vi "test_response string.vi"(8 "error in (no error)":errorcluster, 11 "TestCase in":refnum<class "Return Response Triggers.lvclass">) -> (0 "error out":errorcluster, 3 "TestCase out":refnum<class "Return Response Triggers.lvclass">)   [LabVIEW 2017, in "Return Response Triggers.lvclass"]
uses:
  Return Response Triggers.lvclass
  Libraries/SSH/Return Request Configuration.ctl
  Libraries/SSH/Response Configuration.ctl
  Libraries/SSH/Expected Response String Config.ctl
  <vilib>/addons/_JKI Toolkits/VI Tester/TestCase.llb/TestCase.lvclass
  Libraries/SSH/SSH.lvlib
  C:/Program Files (x86)/National Instruments/LabVIEW 2017/vi.lib/addons/_JKI Toolkits/VI Tester/TestCase.llb/TestCase.lvclass
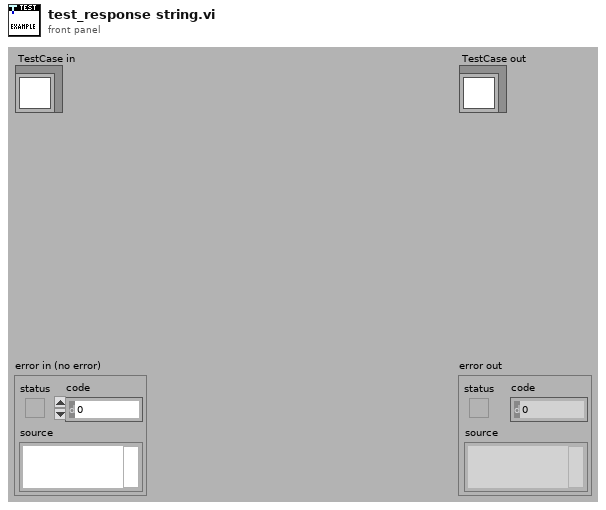
[diagram p1: front panel]
types:
  T1 = typedef "SSH.lvlib/Return Request Configuration.ctl" = cluster{"Response Configuration":T2, "Return Notifier":refnum<notifier>, "Response Requested":bool, "Command":string, "Initial Timer Value":u32}
  T2 = typedef "SSH.lvlib/Response Configuration.ctl" = cluster{"Expected Response String":T3, "Character Count Limit":i32, "Timeout (ms)":i32}
  T3 = typedef "SSH.lvlib/Expected Response String Config.ctl" = cluster{"Expected Response":string, "Search Start Point":enum16{"From Start", "From End"}, "Instance Count":i32}
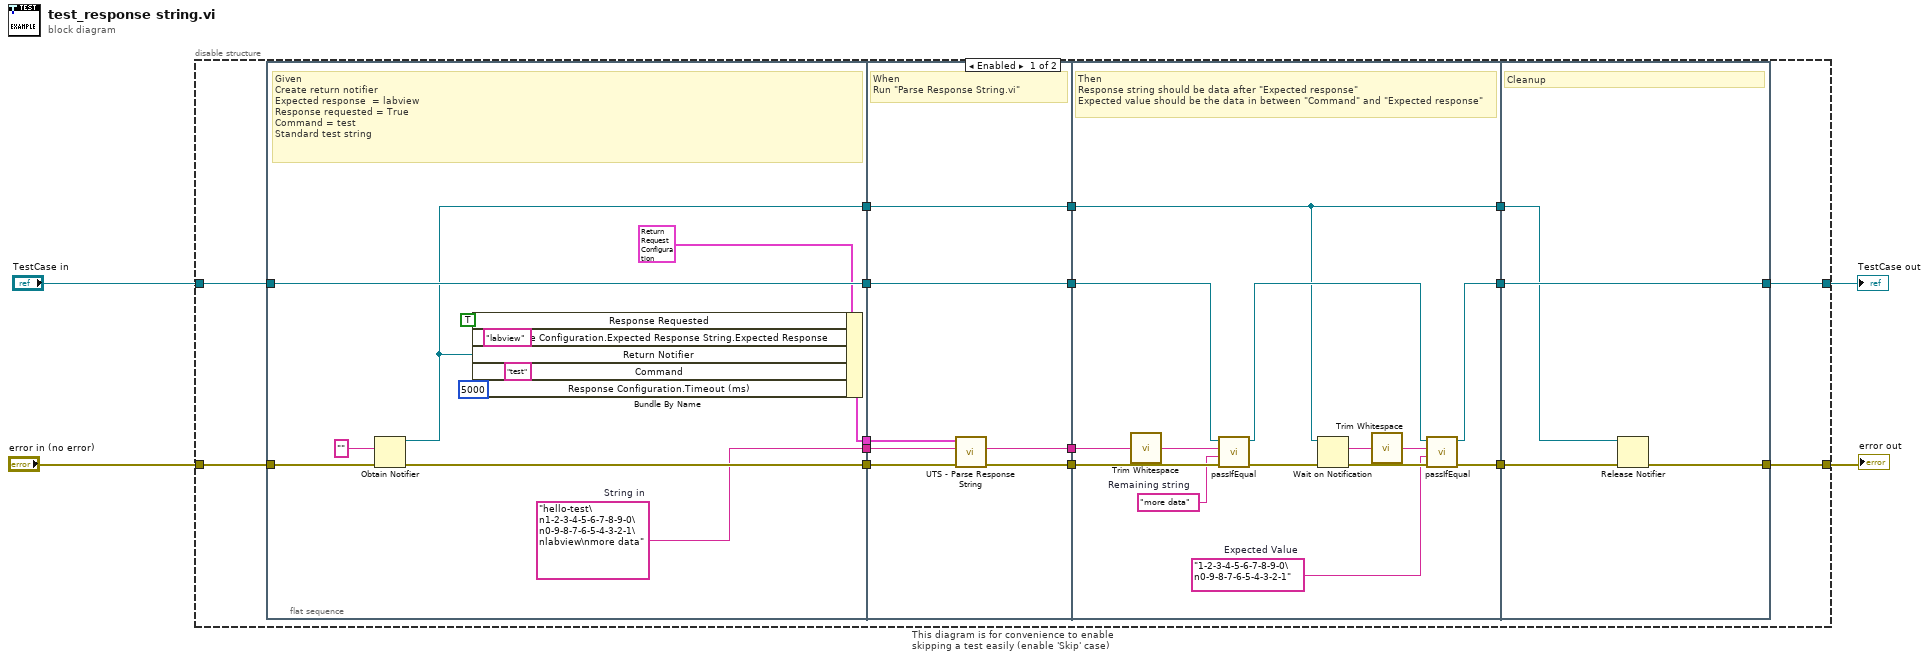
[diagram p0: block diagram]
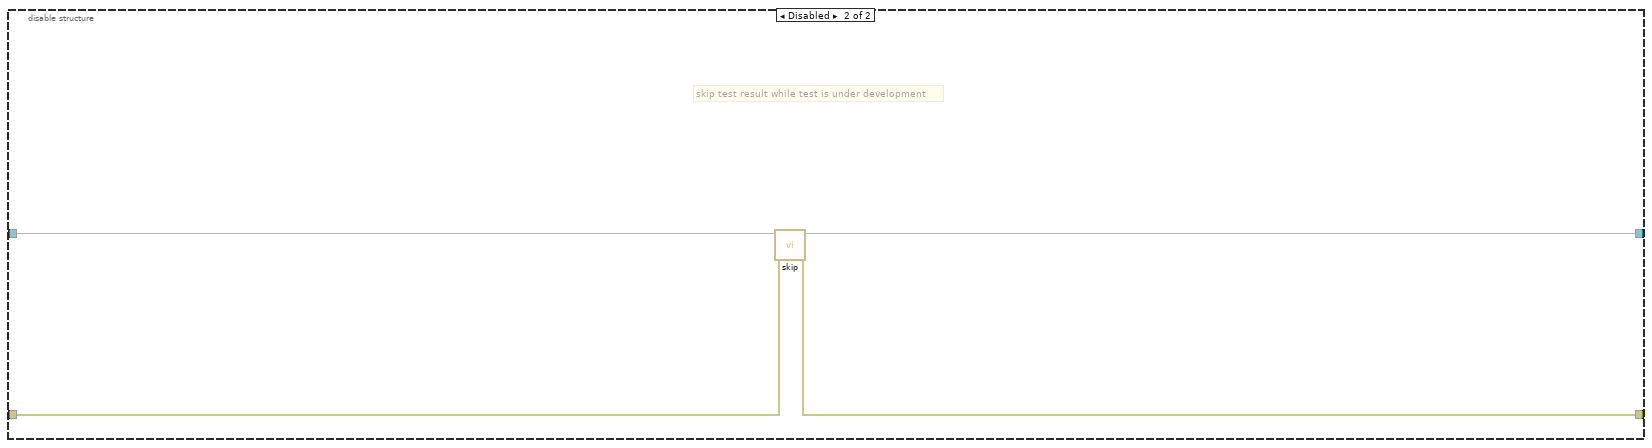
[diagram p2: hidden frame]
diagram:
  n1 = disable-structure "This diagram is for convenience to enable skipping a test easily (enable 'Skip' case)" shown="Enabled" {
    disable-tunnel: "TestCase in" -> [w13 w61]
    disable-tunnel: [w12 w59] -> w1
    disable-tunnel: [w11 w60] -> w3
    disable-tunnel: "error in (no error)" -> [w14 w58]
    frame Enabled {
      n2 = flat-sequence {
        tunnel: w14 -> [w29]
        tunnel: w13 -> [w32]
        tunnel: [w32] -> w20
        tunnel: [w28] -> w19
        tunnel: [w27] -> w10
        tunnel: [w23] -> w9
        tunnel: [w22] -> w8
        tunnel: [w39] -> w18
        tunnel: [w37] -> w17
        tunnel: w20 -> [w39]
        tunnel: w19 -> [w38]
        tunnel: w10 -> [w36]
        tunnel: w9 -> [w33]
        tunnel: w8 -> [w35]
        tunnel: [w34] -> w7
        tunnel: [w33] -> w6
        tunnel: [w46] -> w16
        tunnel: [w48] -> w15
        tunnel: w18 -> [w53]
        tunnel: w17 -> [w52]
        tunnel: w7 -> [w50]
        tunnel: w6 -> [w43]
        tunnel: [w43] -> w5
        tunnel: [w55] -> w11
        tunnel: [w57] -> w12
        tunnel: w16 -> [w57]
        tunnel: w15 -> [w56]
        tunnel: w5 -> [w54]
        frame #0 {
          w22 = "hello-test\n1-2-3-4-5-6-7-8-9-0\n0-9-8-7-6-5-4-3-2-1\nlabview\nmore data"  # String in
          # "Given\nCreate return notifier\nExpected response  = labview\nResponse requested = True\nCommand = test\nStandard test string"
          n3 = Obtain Notifier(notification data type="", error in (no error)=w29) -> (notifier out=w23:refnum<notifier>, error out=w28:errorcluster)  [unwired: 2 in, 1 out]
          n4 = Bundle By Name(cluster=T1 {"Response Configuration"={"Expected Response String"={"Expected Response"="", "Search Start Point"=enum."From Start", "Instance Count"=0}, "Character Count Limit"=0, "Timeout (ms)"=0}, "Return Notifier"=refnum, "Response Requested"=FALSE, "Command"="", "Initial Timer Value"=0} ("Return Request in"), "Response Requested"=TRUE, "Response Configuration.Expected Response String.Expected Response"="labview" ("Response Configuration.Expected Response"), "Return Notifier"=w23, "Command"="test", "Response Configuration.Timeout (ms)"=u32 5000) -> (w27:T1)
        }
        frame #1 {
          # "When\nRun \"Parse Response String.vi\""
          n5 = call "UTS - Parse Response String.vi"("error in (no error)"=w38, "Response String in"=w35, "Return Request in"=w36) -> ("error out"=w37:errorcluster, "Response String out"=w34:string)  [unwired: 6 in, 1 out]
        }
        frame #2 {
          w42 = "more data"  # Remaining string
          w45 = "1-2-3-4-5-6-7-8-9-0\n0-9-8-7-6-5-4-3-2-1"  # Expected Value
          # "Then\nResponse string should be data after \"Expected response\"\nExpected value should be the data in between \"Command\" and \"Expected response\""
          n6 = call <vilib>:"Trim Whitespace.vi"("string"=w50) -> ("trimmed string"=w41:string)  [unwired: 1 in]
          n7 = call-dynamic "passIfEqual.vi"("error in (no error)"=w52, "y"=w42, "x"=w41, "TestCase in"=w53) -> ("error out"=w51:errorcluster, "TestCase out"=w47:refnum<class "Return Response Triggers.lvclass">)  [unwired: 6 in]
          n8 = Wait on Notification(notifier=w43, error in (no error)=w51) -> (notification=w44:string, error out=w49:errorcluster)  [unwired: 2 in, 2 out]
          n9 = call <vilib>:"Trim Whitespace.vi"("string"=w44) -> ("trimmed string"=w40:string)  [unwired: 1 in]
          n10 = call-dynamic "passIfEqual.vi"("error in (no error)"=w49, "y"=w45, "x"=w40, "TestCase in"=w47) -> ("error out"=w48:errorcluster, "TestCase out"=w46:refnum<class "Return Response Triggers.lvclass">)  [unwired: 6 in]
        }
        frame #3 {
          # "Cleanup"
          n11 = Release Notifier(notifier=w54, error in (no error)=w56) -> (error out=w55:errorcluster)  [unwired: 1 in, 2 out]
        }
      }
    }
    frame Disabled {
      # "skip test result while test is under development"
      n12 = call <vilib>:"skip.vi"("error in (no error)"=w58, "TestCase in"=w61) -> ("error out"=w60:errorcluster, "TestCase out"=w59:refnum<class "Return Response Triggers.lvclass">)  [unwired: 8 in]
    }
  }
  "error out" <- w3
  "TestCase out" <- w1
